vi "Convert Timestamp.vi"(10 "Timestamp precision":T1, 11 "Time Stamp":timestamp format="%<%x %.3X>T") -> (3 "Timestamp String":string)   [LabVIEW 2020, in "InfluxDB v2 Client.lvlib"]
doc: "Converts the timestamp to a specific precision"
uses:
  InfluxDB v2 Client.lvlib
  Timestamp precision.ctl
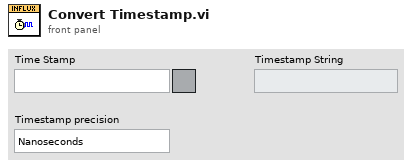
[diagram p1: front panel]
types:
  T1 = typedef "InfluxDB v2 Client.lvlib/Timestamp precision.ctl" = enum16{"Nanoseconds", "Microseconds", "Milliseconds", "Seconds"}
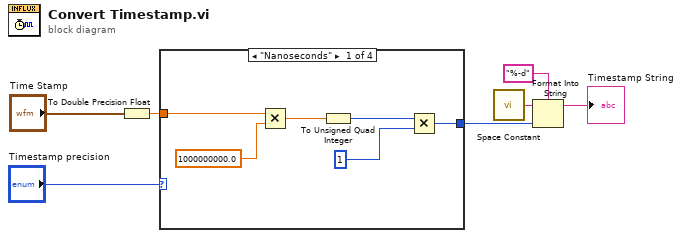
[diagram p0: block diagram]
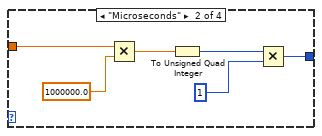
[diagram p2: hidden frame]
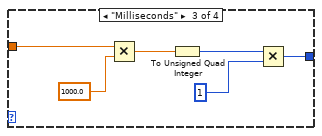
[diagram p3: hidden frame]
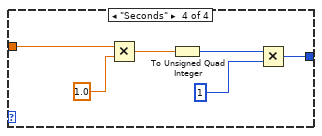
[diagram p4: hidden frame]
diagram:
  n1 = To Double Precision Float(number="Time Stamp") -> (double precision float=w5:dbl)
  n2 = case shown="\"Nanoseconds\"" "Timestamp precision" {
    tunnel: w5 -> [w13 w19 w25 w31]
    tunnel: [w8 w14 w20 w26] -> w7
    frame "Nanoseconds" {
      n3 = Multiply(x=w13, y=1000000000.0) -> (x*y=w11:dbl)
      n4 = To Unsigned Quad Integer(1:w11) -> (0:w10:u64)
      n5 = Multiply(x=w10, y=u64 1) -> (x*y=w8:u64)
    }
    frame "Microseconds" {
      n6 = Multiply(x=w19, y=1000000.0) -> (x*y=w17:dbl)
      n7 = To Unsigned Quad Integer(1:w17) -> (0:w16:u64)
      n8 = Multiply(x=w16, y=u64 1) -> (x*y=w14:u64)
    }
    frame "Milliseconds" {
      n9 = Multiply(x=w25, y=1000.0) -> (x*y=w23:dbl)
      n10 = To Unsigned Quad Integer(1:w23) -> (0:w22:u64)
      n11 = Multiply(x=w22, y=u64 1) -> (x*y=w20:u64)
    }
    frame "Seconds" {
      n12 = Multiply(x=w31, y=1.0) -> (x*y=w29:dbl)
      n13 = To Unsigned Quad Integer(1:w29) -> (0:w28:u64)
      n14 = Multiply(x=w28, y=u64 1) -> (x*y=w26:u64)
    }
  }
  n15 = call <vilib>:"Space Constant.vi"() -> ("String"=w6:string)
  n16 = Format Into String(format string="%-d", initial string=w6, w7) -> (resulting string=→"Timestamp String":string)  [unwired: 1 in, 1 out]
